vi "JSONToParam.vi"(8 "error in":errorcluster, 10 "JSON":string, 11 "paramUnicornIn":T1={"conParam"={"ReadIntParam"=TRUE, "ReadDescrParam"=FALSE, "ReadFloatParam"=TRUE, "debug"=FALSE, "ReadJSON"=TRUE, "IP_address"="192.168.1.216", "N_attempts"=3, "type_con"=enum."TCP", "MB_address"=1, "VISA"="COM1", "connection ID"=refnum, "nameDevices"="", "timeout"=3000, "port"=2000, "type_version"="0F0C0001", "baud_rate"=115200, "VersionControl"=TRUE, "TCP_conn"=TRUE, "WindowSize"=700}, "Param"={"NumParam"={"NTelem"=201, "NInt"=16, "NFloat"=10, "NTable"=2}, "ParamInt"=[{"ID"="Режим работы", "Num"=0, "Name"="", "Type"="", "Enum"="", "Desc"="", "Unit"="", "Access"="", "FormatStr"="", "Min"=0, "Max"=0}, {"ID"="", "Num"=0, "Name"="", "Type"="", "Enum"="", "Desc"="", "Unit"="", "Access"="", "FormatStr"="", "Min"=0, "Max"=0}, {"ID"="", "Num"=0, "Name"="", "Type"="", "Enum"="", "Desc"="", "Unit"="", "Access"="", "FormatStr"="", "Min"=0, "Max"=0}, {"ID"="", "Num"=0, "Name"="", "Type"="", "Enum"="", "Desc"="", "Unit"="", "Access"="", "FormatStr"="", "Min"=0, "Max"=0}, {"ID"="", "Num"=0, "Name"="", "Type"="", "Enum"="", "Desc"="", "Unit"="", "Access"="", "FormatStr"="", "Min"=0, "Max"=0}, {"ID"="", "Num"=0, "Name"="", "Type"="", "Enum"="", "Desc"="", "Unit"="", "Access"="", "FormatStr"="", "Min"=0, "Max"=0}, {"ID"="ModeWork", "Num"=0, "Name"="", "Type"="", "Enum"="", "Desc"="", "Unit"="", "Access"="", "FormatStr"="", "Min"=0, "Max"=0}], "Telemetry"=[], "Table"=[], "ParamFloat"=[]}}) -> (0 "error out":errorcluster, 3 "paramUnicornOut":T1={"conParam"={"ReadIntParam"=TRUE, "ReadDescrParam"=FALSE, "ReadFloatParam"=TRUE, "debug"=FALSE, "ReadJSON"=TRUE, "IP_address"="192.168.1.216", "N_attempts"=3, "type_con"=enum."TCP", "MB_address"=1, "VISA"="COM1", "connection ID"=refnum, "nameDevices"="", "timeout"=3000, "port"=2000, "type_version"="0F0C0001", "baud_rate"=115200, "VersionControl"=TRUE, "TCP_conn"=TRUE, "WindowSize"=700}, "Param"={"NumParam"={"NTelem"=201, "NInt"=16, "NFloat"=10, "NTable"=2}, "ParamInt"=[], "Telemetry"=[], "Table"=[], "ParamFloat"=[]}})   [LabVIEW 2017, in "LV_Unicorn.lvlib"]
uses:
  LV_Unicorn.lvlib
  Control/unicorn_Param.ctl
  Control/unicorn_conn.ctl
  Control/unicorn_JSON.ctl
  Control/unicorn_ParamInt.ctl
  Control/unicorn_Telemetry.ctl
  Control/unicorn_Table.ctl
  Control/unicorn_ParamFloat.ctl
  8ed377cf-5d0a-4df8-8753-8aee4b7220c6.vi
  0a05eefe-cb57-45bc-8247-07be7b8f4c8f.vi
  59de7177-ab15-4b4d-9abb-16a12f5f9711.vi
  00bf21b9-44ad-4b67-ade8-f11928027645.vi
  <vilib>/JDP Science/JSONtext/Next JSON Value.vi
  <vilib>/JDP Science/JSONtext/String Subset.vi
  <vilib>/JDP Science/JSONtext/Parsing/Advance past next JSON Value (inlined COPY).vi
  <vilib>/JDP Science/JSONtext/Parsing/Advance past whitespace.vi
  <vilib>/JDP Science/JSONtext/Parsing/Advance past String.vi
  <vilib>/JDP Science/JSONtext/Parsing/Advance past Number.vi
  <vilib>/JDP Science/JSONtext/Parsing/Advance past Line Ending.vi
  <vilib>/JDP Science/JSONtext/Parsing/Parse Full Path or Item Name.vi
  <vilib>/JDP Science/JSONtext/Parsing/Advance past Array.vi
  <vilib>/JDP Science/JSONtext/Parsing/Advance past Object.vi
  <vilib>/JDP Science/JSONtext/support/Error Cluster From Code.vi
  <vilib>/JDP Science/JSONtext/Offset/Find Item Locations by Path.vi
  <vilib>/JDP Science/JSONtext/JSON text to Variant.vi
  <vilib>/JDP Science/JSONtext/LVClass Serializer/JSONtext LVClass Serializer.lvclass
  <vilib>/JDP Science/JSONtext/JSONtext.lvlib
  <vilib>/addons/Tools/Unicode/UTF8 Tools.lvlib
panel:
  out "Rest of Input String":string
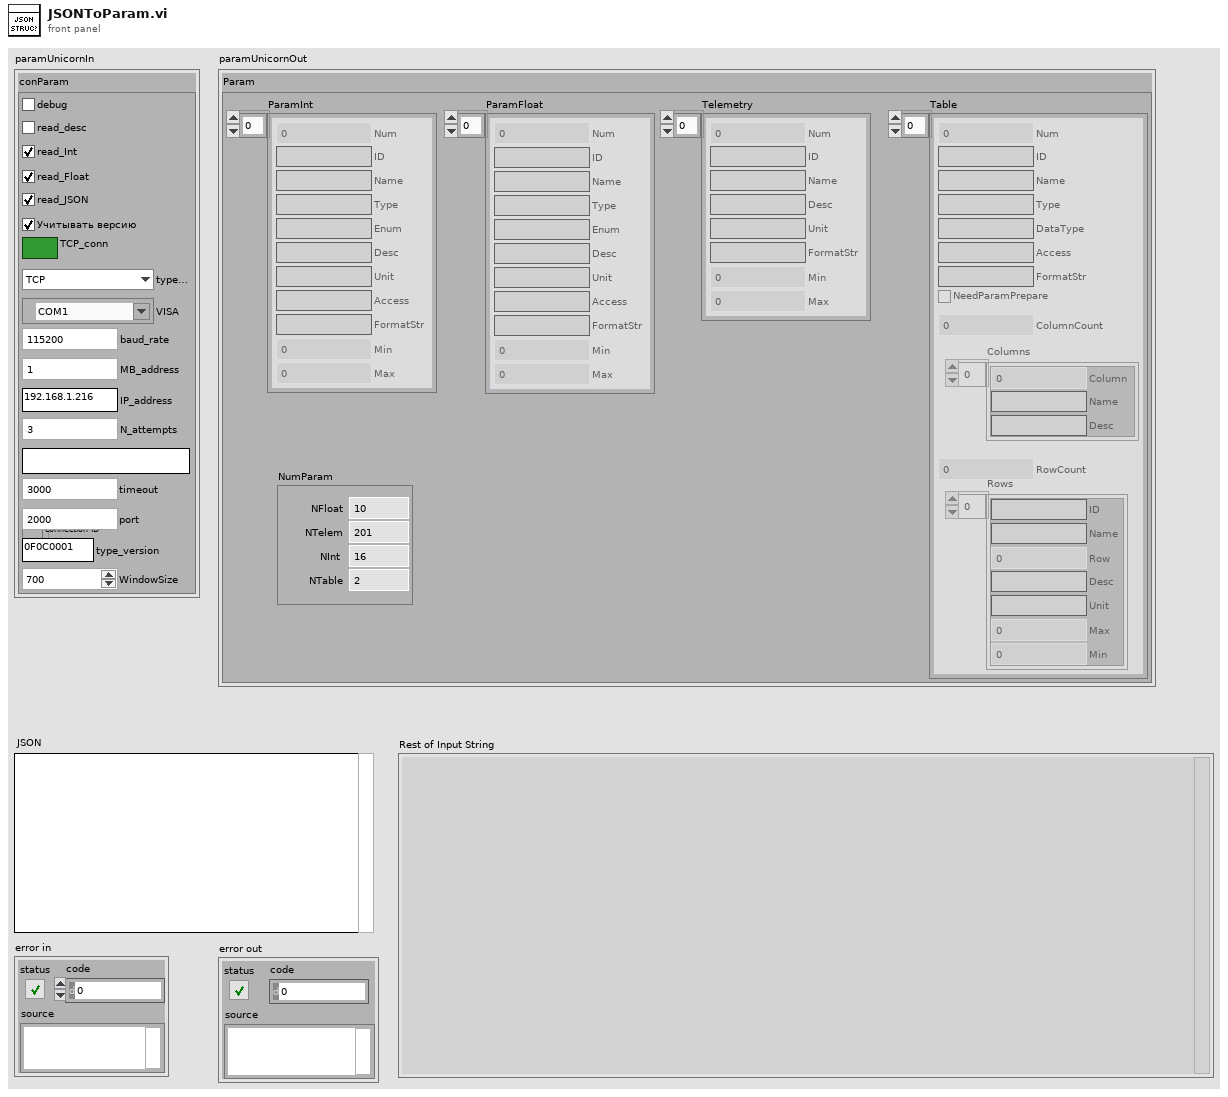
[diagram p1: front panel]
types:
  T1 = typedef "LV_Unicorn.lvlib/unicorn_Param.ctl" = cluster{"conParam":T2, "Param":T3}
  T2 = typedef "LV_Unicorn.lvlib/unicorn_conn.ctl" = cluster{"ReadIntParam":bool, "ReadDescrParam":bool, "ReadFloatParam":bool, "debug":bool, "ReadJSON":bool, "IP_address":string, "N_attempts":i32, "type_con":enum16{"Serial", "TCP"}, "MB_address":i32, "VISA":refnum<visa-resource-name>, "connection ID":refnum<k5>, "nameDevices":string, "timeout":i32, "port":u16, "type_version":string, "baud_rate":u32, "VersionControl":bool, "TCP_conn":bool, "WindowSize":i32}
  T3 = typedef "LV_Unicorn.lvlib/unicorn_JSON.ctl" = cluster{"NumParam":cluster{"NTelem":i32, "NInt":i32, "NFloat":i32, "NTable":i32}, "ParamInt":T4, "Telemetry":T5, "Table":T6, "ParamFloat":T7}
  T4 = typedef "LV_Unicorn.lvlib/unicorn_ParamInt.ctl" = cluster{"ID":string, "Num":i32, "Name":string, "Type":string, "Enum":string, "Desc":string, "Unit":string, "Access":string, "FormatStr":string, "Min":i32, "Max":i32}[]
  T5 = typedef "LV_Unicorn.lvlib/unicorn_Telemetry.ctl" = cluster{"ID":string, "Num":i32, "Name":string, "Desc":string, "Unit":string, "FormatStr":string, "Min":i32, "Max":i32}[]
  T6 = typedef "LV_Unicorn.lvlib/unicorn_Table.ctl" = cluster{"Num":i32, "Access":string, "ColumnCount":i32, "NeedParamPrepare":bool, "Columns":cluster{"Column":i32, "Desc":string, "Name":string}[], "DataType":string, "FormatStr":string, "ID":string, "Name":string, "RowCount":i32, "Rows":cluster{"Desc":string, "ID":string, "Max":i32, "Min":i32, "Name":string, "Row":i32, "Unit":string}[], "Type":string}[]
  T7 = typedef "LV_Unicorn.lvlib/unicorn_ParamFloat.ctl" = cluster{"ID":string, "Num":i32, "Name":string, "Type":string, "Enum":string, "Desc":string, "Unit":string, "Access":string, "FormatStr":string, "Min":sgl, "Max":sgl}[]
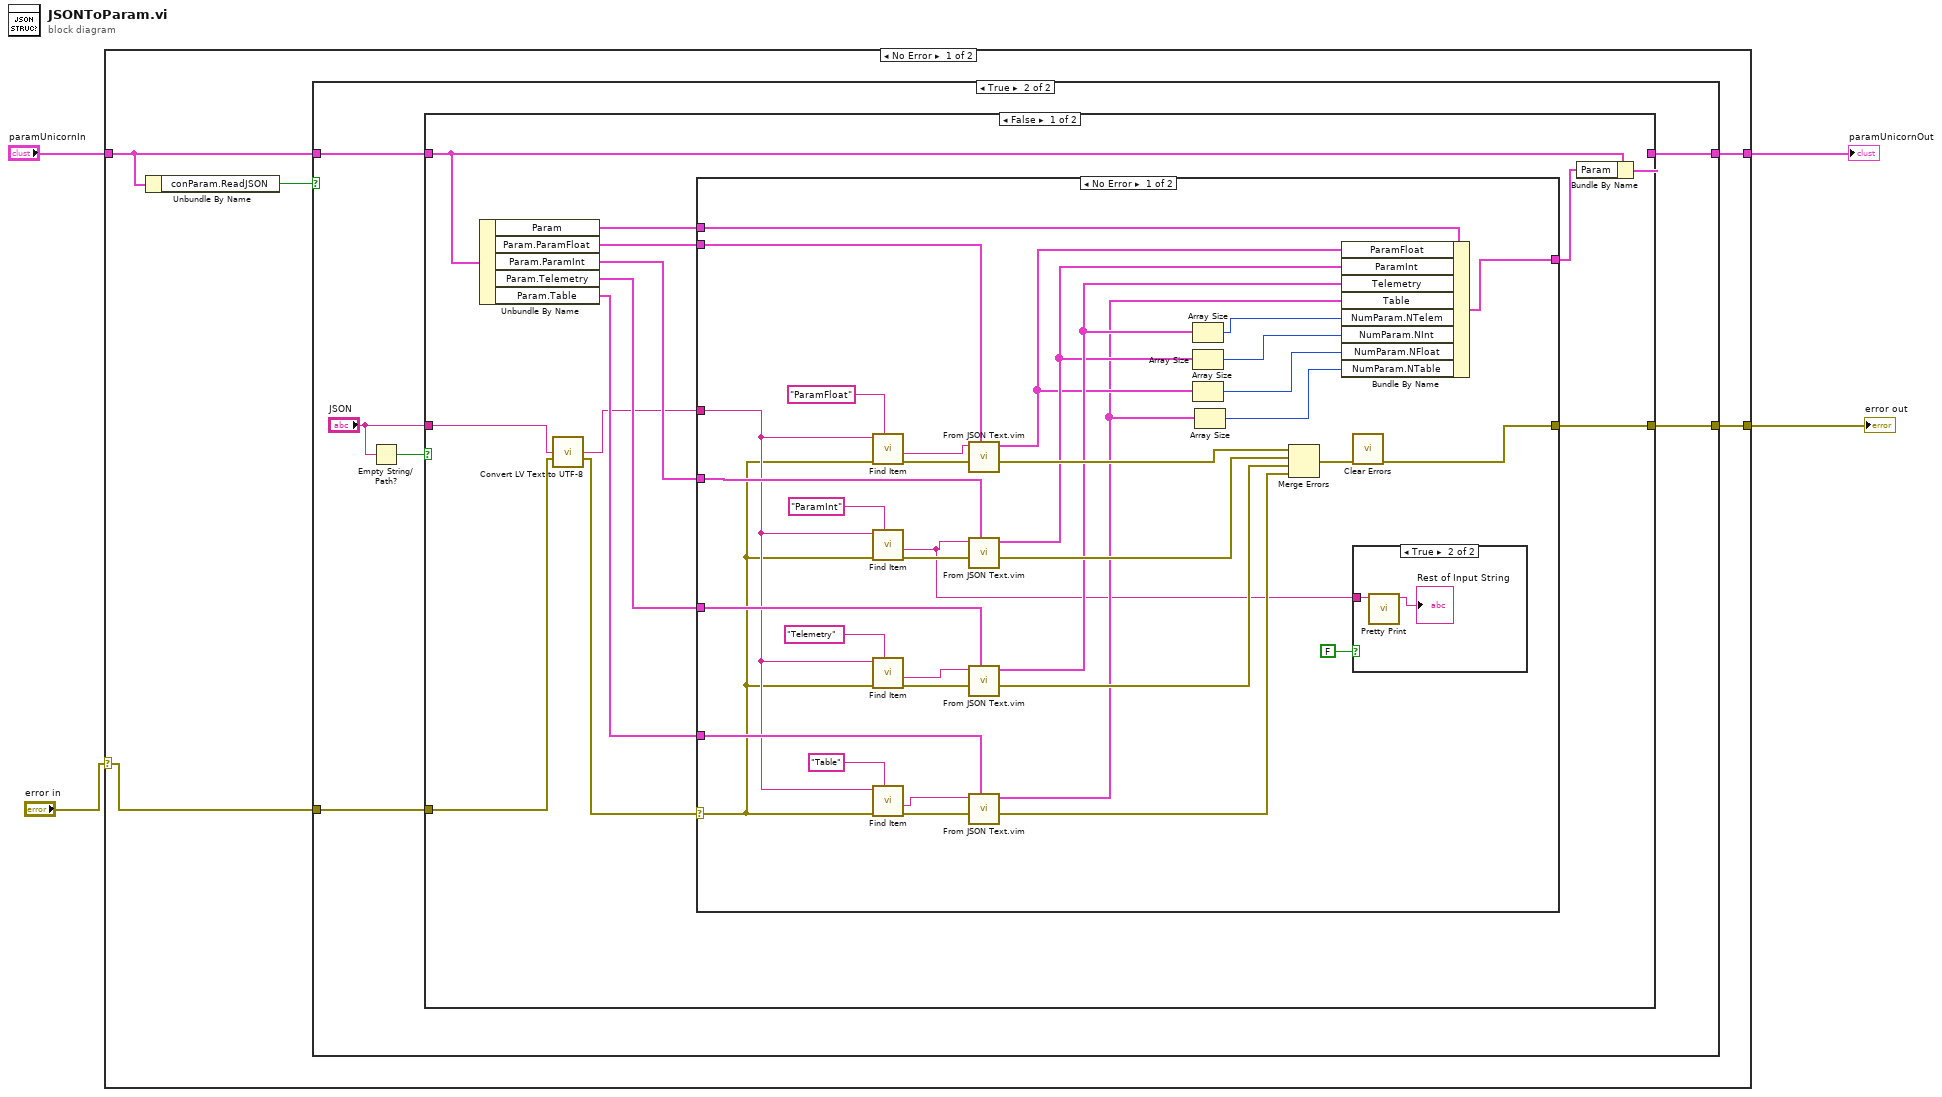
[diagram p0: block diagram]
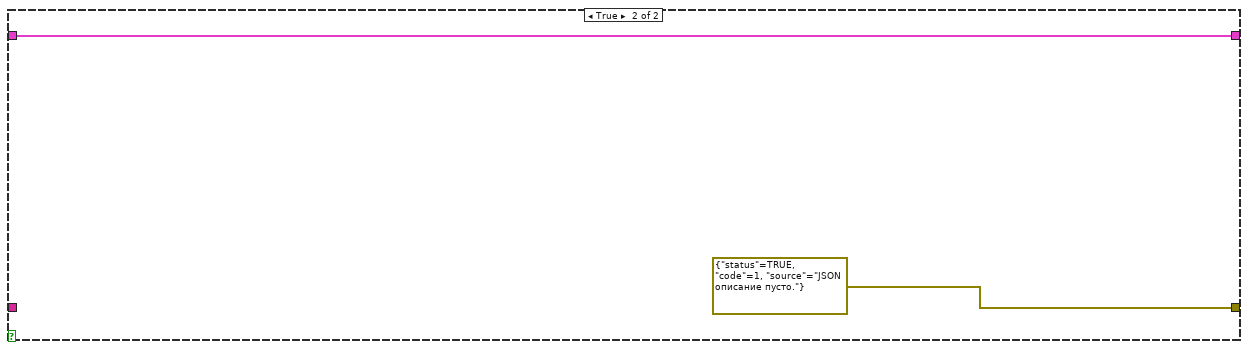
[diagram p5: hidden frame]
diagram:
  n1 = case shown="No Error" "error in" {
    selector: "error in" -> [w5 w72]
    tunnel: [w9 w73] -> w4
    tunnel: [w8 w72] -> w3
    tunnel: "paramUnicornIn" -> [w7 w73]
    frame No Error {
      n2 = Unbundle By Name(w7) -> ("conParam.ReadJSON"=w6:bool)
      n3 = case shown="True" w6 {
        tunnel: [w11 w17] -> w9
        tunnel: w5 -> [w10 w16]
        tunnel: [w10 w13] -> w8
        tunnel: w7 -> [w11 w12]
        frame False {
        }
        frame True {
          n4 = Empty String/Path?(string/path="JSON") -> (empty?=w14:bool)
          n5 = case shown="False" w14 {
            tunnel: w12 -> [w30 w71]
            tunnel: [w28 w71] -> w17
            tunnel: w16 -> [w21 _]
            tunnel: "JSON" -> [w19 _]
            tunnel: [w18 errorcluster {"status"=TRUE, "code"=1, "source"="JSON описание пусто."} ("error IO")] -> w13
            frame False {
              n6 = Unbundle By Name(w30) -> ("Param"=w23:T3, "Param.ParamFloat"=w22:T7, "Param.ParamInt"=w25:T4, "Param.Telemetry"=w26:T5, "Param.Table"=w27:T6)
              n7 = call <vilib>:"Convert LV Text to UTF-8.vi"("LV Text"=w19, "error in"=w21) -> ("UTF-8 Text"=w24:string, "error out"=w20:errorcluster)  [unwired: 12 in]
              n8 = case shown="No Error" w20 {
                selector: w20 -> [w47 w69]
                tunnel: w24 -> [w48 _]
                tunnel: [w31 w69] -> w18
                tunnel: w23 -> [w64 w68]
                tunnel: [w63 w68] -> w29
                tunnel: w27 -> [w51 _]
                tunnel: w26 -> [w56 _]
                tunnel: w25 -> [w60 _]
                tunnel: w22 -> [w44 _]
                frame No Error {
                  n9 = call <vilib>:"Find Item.vi"("$Path or Item Name"="ParamFloat", "error in (no error)"=w47, "JSON"=w48) -> ("error out"=w46:errorcluster, "<JSON>"=w45:string)  [unwired: 5 in, 2 out]
                  n10 = call <vilib>:"Find Item.vi"("$Path or Item Name"="ParamInt", "error in (no error)"=w47, "JSON"=w48) -> ("error out"=w58:errorcluster, "<JSON>"=w33:string)  [unwired: 5 in, 2 out]
                  n11 = call <vilib>:"Find Item.vi"("$Path or Item Name"="Telemetry", "error in (no error)"=w47, "JSON"=w48) -> ("error out"=w57:errorcluster, "<JSON>"=w55:string)  [unwired: 5 in, 2 out]
                  n12 = call <vilib>:"Find Item.vi"("$Path or Item Name"="Table", "error in (no error)"=w47, "JSON"=w48) -> ("error out"=w53:errorcluster, "<JSON>"=w52:string)  [unwired: 5 in, 2 out]
                  n13 = call "From JSON Text.vim"("Data Type and Default Value"=w44, "error in (no error)"=w46, "JSON"=w45) -> ("error out"=w43:errorcluster, "Data out"=w38:T7)  [unwired: 7 in]
                  n14 = call "From JSON Text.vim"("Data Type and Default Value"=w60, "error in (no error)"=w58, "JSON"=w33) -> ("error out"=w59:errorcluster, "Data out"=w40:T4)  [unwired: 7 in]
                  n15 = call "From JSON Text.vim"("Data Type and Default Value"=w56, "error in (no error)"=w57, "JSON"=w55) -> ("error out"=w54:errorcluster, "Data out"=w42:T5)  [unwired: 7 in]
                  n16 = call "From JSON Text.vim"("Data Type and Default Value"=w51, "error in (no error)"=w53, "JSON"=w52) -> ("error out"=w50:errorcluster, "Data out"=w36:T6)  [unwired: 7 in]
                  n17 = Array Size(array=w42) -> (size(s)=w41:i32)
                  n18 = Array Size(array=w40) -> (size(s)=w39:i32)
                  n19 = Array Size(array=w38) -> (size(s)=w37:i32)
                  n20 = Array Size(array=w36) -> (size(s)=w35:i32)
                  n21 = Merge Errors(w43, w59, w54, w50) -> (w32:errorcluster)
                  n22 = Bundle By Name(cluster=w64, "ParamFloat"=w38, "ParamInt"=w40, "Telemetry"=w42, "Table"=w36, "NumParam.NTelem"=w41, "NumParam.NInt"=w39, "NumParam.NFloat"=w37, "NumParam.NTable"=w35) -> (w63:T3)
                  n23 = call <vilib>:"Clear Errors.vi"("error in (no error)"=w32) -> ("error out"=w31:errorcluster)  [unwired: 5 in, 1 out]
                  n24 = case shown="True" FALSE {
                    tunnel: w33 -> [_ w67]
                    frame False {
                    }
                    frame True {
                      n25 = call <vilib>:"Pretty Print.vi"("JSON"=w67) -> ("<JSON>"=→"Rest of Input String":string)  [unwired: 8 in, 2 out]
                    }
                  }
                }
                frame Error {
                }
              }
              n26 = Bundle By Name(cluster=w30, "Param"=w29) -> (w28:T1)
            }
            frame True {
            }
          }
        }
      }
    }
    frame Error {
    }
  }
  "paramUnicornOut" <- w4
  "error out" <- w3
